vi "Hierarchy To Build Order Recursive.vi"(0 "Working Set":refnum<data-value>, 11 "error in (no error)":errorcluster) -> (4 "Exports":refnum<class "Export.lvclass">[](array[class]), 15 "error out":errorcluster)   [LabVIEW 2017, in "CL_G3_VIComponentBuilder.lvlib" / "Build Analyzer.lvclass"]
doc: "Translates either a Dependency (top down) or Dependant (bubble up) hierarchy to a build order of exports."
uses:
  Build Analyzer.lvclass
  Exports/Exports/Export.lvclass
  <userlib>/_Cirrus Logic/LabVIEW Container/Source/Container/Container.lvclass
  <userlib>/_Cirrus Logic/LabVIEW Container/Source/Container/Container.lvclass/Container.ctl
  <userlib>/_Cirrus Logic/LabVIEW Container/Source/Container/GetAttribute_Variant.vi
  <userlib>/_Cirrus Logic/LabVIEW Container/Source/Container/SubVIs/GetAttribute_ByValue.vi
  <userlib>/_Cirrus Logic/LabVIEW Container/Source/Container/Get All Children.vi
  <userlib>/_Cirrus Logic/LabVIEW Container/Source/CIR/Interface Definition/Container Intermediate Representation.lvclass
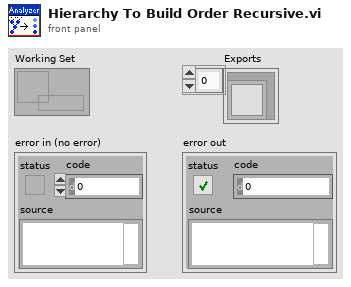
[diagram p1: front panel]
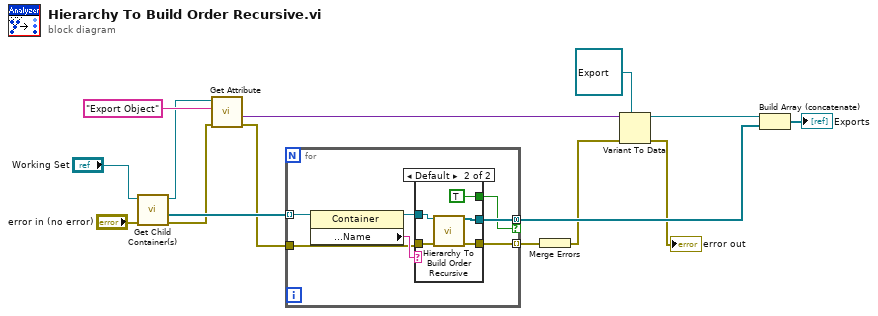
[diagram p0: block diagram]
diagram:
  n1 = call-poly <userlib>:"Get Child Container(s).vi"("error in (no error)"="error in (no error)", "Container"="Working Set") -> ("error out"=w5:errorcluster, "Child Containers"=w13:refnum<data-value>[], "dup Container"=w14:refnum<data-value>)  [unwired: 6 in, 1 out]
  n2 = call-poly <userlib>:"Get Attribute.vi"("error in (no error)"=w5, "Attribute Name"="Export Object", "Container Reference in"=w14) -> ("error out"=w4:errorcluster, "Attribute Value"=w12:variant)  [unwired: 5 in, 2 out]
  n3 = for {
    tunnel: w13 -> [w21] mode=indexing
    tunnel: [w22] -> w9 mode=concatenating if=w19
    tunnel: w4 -> [w18]
    tunnel: [w17] -> w2 mode=indexing
    n4 = property class="Container"(reference=w21) -> (reference out=w16:refnum<data-value>, "Palette VIs:Property Definitions:Name"=w20:string)  [unwired: 1 in, 1 out]
    n5 = case shown="Default" w20 {
      tunnel: [_ w28] -> w22
      tunnel: w16 -> [_ w27]
      tunnel: [_ TRUE] -> w19
      tunnel: w18 -> [w23 w25]
      tunnel: [w23 w24] -> w17
      frame "Dependency Unique VI Package Names" {
      }
      frame Default {
        n6 = call "Hierarchy To Build Order Recursive.vi"("Working Set"=w27, "error in (no error)"=w25) -> ("Exports"=w28:refnum<class "Export.lvclass">[], "error out"=w24:errorcluster)  [unwired: 12 in]
      }
    }
  }
  n7 = Merge Errors(w2) -> (w1:errorcluster)
  n8 = Variant To Data(error in=w1, type=refnum<class "Export.lvclass"> refnum ("Export Out"), Variant=w12) -> (data=w11:refnum<class "Export.lvclass">, error out=→"error out":errorcluster)
  n9 = Build Array (concatenate)(w11, w9) -> (→"Exports":refnum<class "Export.lvclass">[])
